vi "Get UUT Info.vi"(0 "reference in":refnum<class "UUT.lvclass">, 7 "error in (no error)":errorcluster) -> (17 "Pull Position (mm)":dbl, 18 "UUT Info All":T1, 19 "Push Position (mm)":dbl, 20 "reference out":refnum<class "UUT.lvclass">, 21 "Part Number":string, 22 "Lower Push Limit (lb)":dbl, 23 "Upper Push Limit (lb)":dbl, 24 "Lower Pull Limit (lb)":dbl, 25 "Upper Pull Limit (lb)":dbl, 27 "error out":errorcluster)   [LabVIEW 2017, in "UUT.lvclass"]
uses:
  UUT.lvclass
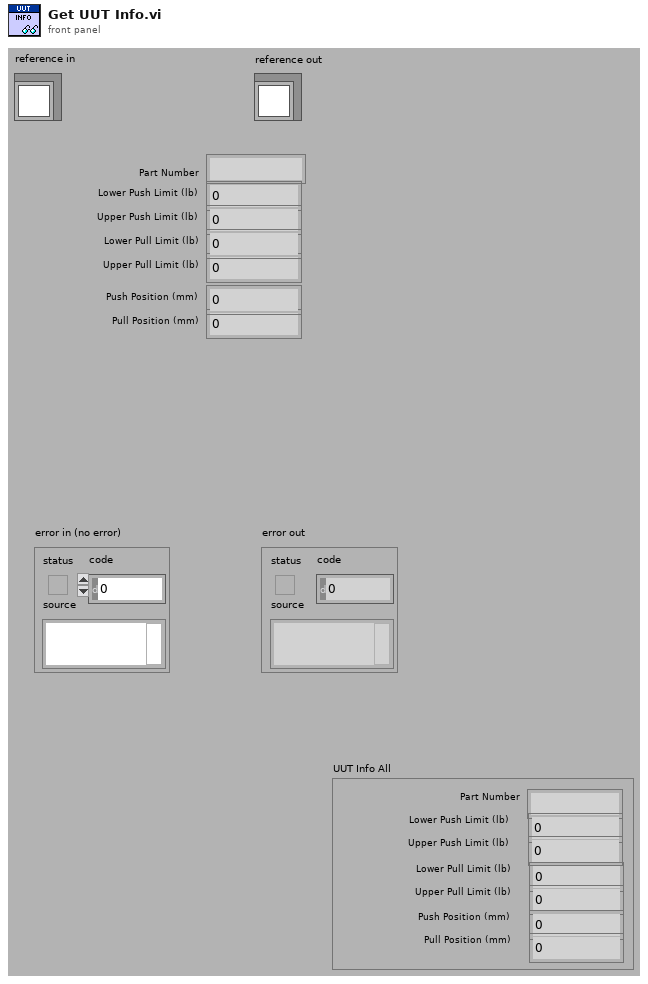
[diagram p1: front panel]
types:
  T1 = cluster{"Part Number":string, "Lower Push Limit (lb)":dbl, "Upper Push Limit (lb)":dbl, "Lower Pull Limit (lb)":dbl, "Upper Pull Limit (lb)":dbl, "Push Position (mm)":dbl, "Pull Position (mm)":dbl}
  T2 = typedef "UUT.lvclass/ObjectAttributes.ctl" = cluster{"UUT Info":cluster{"Part Number":string, "Lower Push Limit (lb)":dbl, "Upper Push Limit (lb)":dbl, "Lower Pull Limit (lb)":dbl, "Upper Pull Limit (lb)":dbl, "Push Position (mm)":dbl, "Pull Position (mm)":dbl}, "Test Results":cluster{"Test Time":timestamp, "Number of Trials":u32, "Push Values (lb)":dbl[], "Push Average (lb)":dbl, "Push Std Dev (lb)":dbl, "Push Passed":bool, "Pull Values (lb)":dbl[], "Pull Average (lb)":dbl, "Pull Std Dev (lb)":dbl, "Pull Passed":bool}}
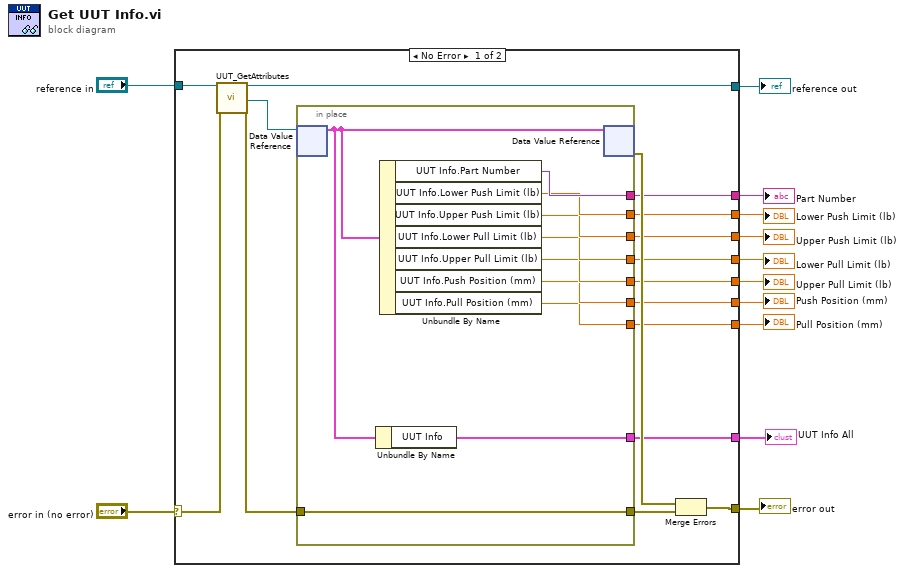
[diagram p0: block diagram]
diagram:
  n1 = case shown="No Error" "error in (no error)" {
    selector: "error in (no error)" -> [w27 w40]
    tunnel: [w25 w40] -> w11
    tunnel: [w26 w39] -> w9
    tunnel: "reference in" -> [w28 w39]
    tunnel: [w20 _] -> w8
    tunnel: [w19 _] -> w7
    tunnel: [w18 _] -> w6
    tunnel: [w17 _] -> w5
    tunnel: [w16 _] -> w4
    tunnel: [w15 _] -> w3
    tunnel: [w14 _] -> w2
    tunnel: [w13 _] -> w1
    frame No Error {
      n2 = call "UUT_GetAttributes.vi"("reference in"=w28, "error in (no error)"=w27) -> ("reference out"=w26:refnum<class "UUT.lvclass">, "DataRef"=w24:refnum<data-value>, "error out"=w23:errorcluster)  [unwired: 14 in, 1 out]
      n3 = in-place {
        in-place-border: w23 -> [w38]
        in-place-border: [w38] -> w22
        in-place-border: [w37] -> w20
        in-place-border: [w36] -> w19
        in-place-border: [w35] -> w18
        in-place-border: [w34] -> w17
        in-place-border: [w33] -> w16
        in-place-border: [w32] -> w15
        in-place-border: [w31] -> w14
        in-place-border: [w29] -> w13
        n4 = in-place-dvr #1(w24) -> (w30:T2)  [unwired: 1 out]
        n5 = Unbundle By Name(w30) -> ("UUT Info"=w29:T1)
        n6 = Unbundle By Name(w30) -> ("UUT Info.Part Number"=w37:string, "UUT Info.Lower Push Limit (lb)"=w36:dbl, "UUT Info.Upper Push Limit (lb)"=w35:dbl, "UUT Info.Lower Pull Limit (lb)"=w34:dbl, "UUT Info.Upper Pull Limit (lb)"=w33:dbl, "UUT Info.Push Position (mm)"=w32:dbl, "UUT Info.Pull Position (mm)"=w31:dbl)
        n7 = in-place-dvr #1(w30) -> (w21:errorcluster)  [unwired: 1 out]
      }
      n8 = Merge Errors(w21, w22) -> (w25:errorcluster)
    }
    frame Error {
    }
  }
  "error out" <- w11
  "reference out" <- w9
  "Part Number" <- w8
  "Lower Push Limit (lb)" <- w7
  "Upper Push Limit (lb)" <- w6
  "Lower Pull Limit (lb)" <- w5
  "Upper Pull Limit (lb)" <- w4
  "Push Position (mm)" <- w3
  "Pull Position (mm)" <- w2
  "UUT Info All" <- w1
